vi "Wait Motor 0 RPM (SubVI).vi"(7 "Strin":string, 8 "error in (no error)":errorcluster, 9 "Motor Speed RPM Serial":refnum<vi>, 10 "Pannel User Message":refnum<vi>, 11 "Stop":refnum<vi>) -> (1 "Stopped":bool)   [LabVIEW 2017]
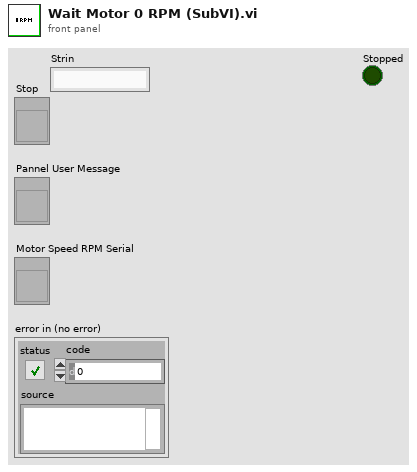
[diagram p1: front panel]
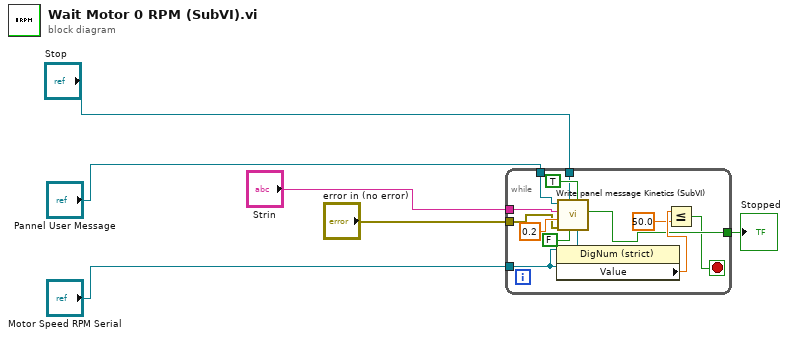
[diagram p0: block diagram]
diagram:
  n1 = while {
    tunnel: "error in (no error)" -> [w15]
    tunnel: "Stop" -> [w14]
    tunnel: "Pannel User Message" -> [w13]
    tunnel: "Motor Speed RPM Serial" -> [w12]
    tunnel: [w9] -> w2
    tunnel: "Strin" -> [w8]
    stop <- w7 stop-if-true
    n2 = property class="DigNum (strict)"(reference=w12) -> ("Value"=w11:dbl)  [unwired: 1 in, 2 out]
    n3 = call "Write panel message Kinetics (SubVI).vi"(4:"rpm"=w12, 5:"rpm"=TRUE ("rpm"), "PrintTime"=FALSE, "Stop"=w14, "error in (no error)"=w15, "Time to wait"=0.2, "Strin"=w8, "String in"=w13) -> ("Stopped"=w9:bool)  [unwired: 1 in, 2 out]
    n4 = Less Or Equal?(x=w11, y=50.0) -> (x <= y?=w7:bool)
  }
  "Stopped" <- w2
